vi "Day 1.vi"() -> ()   [LabVIEW 2020]
uses:
  <vilib>/Utility/file.llb/Read Delimited Spreadsheet (I64).vi
panel:
  out "Increases":i32
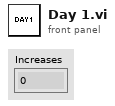
[diagram p1: front panel]
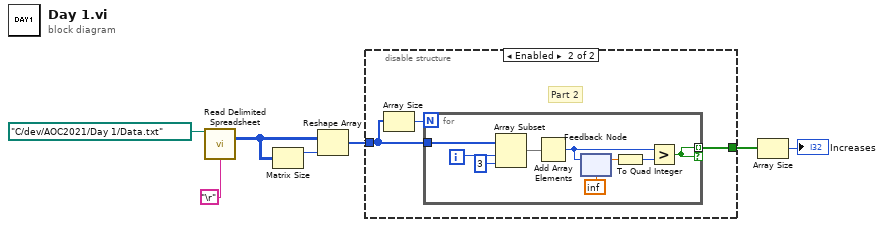
[diagram p0: block diagram]
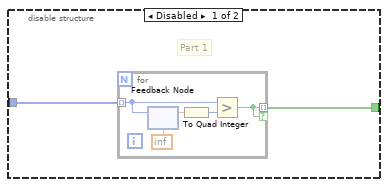
[diagram p2: hidden frame]
diagram:
  n1 = call-poly <vilib>:"Read Delimited Spreadsheet.vi"("file path (dialog if empty)"=path "C:/dev/AOC2021/Day 1/Data.txt", "delimiter (\\t)"="\r" ("delimiter (\\t)")) -> ("all rows"=w5:i64[][])  [unwired: 8 in, 5 out]
  n2 = Matrix Size(0:w5) -> (1:w4:i32)  [unwired: 1 out]
  n3 = Reshape Array(w5, w4) -> (w3:i64[])
  n4 = disable-structure shown="Enabled" {
    disable-tunnel: w3 -> [w9 w15]
    disable-tunnel: [w8 w17] -> w2
    frame Disabled {
      # "Part 1"
      n5 = for {
        tunnel: w9 -> [w13] mode=indexing
        tunnel: [w10] -> w8 mode=indexing if=w10
        n6 = feedback-in #1(w13) -> ()
        n7 = feedback #1(inf) -> (w12:dbl)
        n8 = To Quad Integer(1:w12) -> (0:w11:i64)
        n9 = Greater?(x=w13, y=w11) -> (0:w10:bool)
      }
    }
    frame Enabled {
      # "Part 2"
      n10 = Array Size(array=w15) -> (size(s)=w16:i32)
      n11 = for {
        N: w16 -> [_]
        tunnel: w15 -> [w26]
        tunnel: [w18] -> w17 mode=indexing if=w18
        i -> [w21]
        n12 = Array Subset(array=w26, index=w21, length=3) -> (w20:i64[])
        n13 = Add Array Elements(numeric array=w20) -> (sum=w22:i64)
        n14 = feedback #2(inf) -> (w24:dbl)
        n15 = feedback-in #2(w22) -> ()
        n16 = To Quad Integer(1:w24) -> (0:w23:i64)
        n17 = Greater?(x=w22, y=w23) -> (0:w18:bool)
      }
    }
  }
  n18 = Array Size(array=w2) -> (size(s)=→"Increases":i32)
